vi "Write Name.vi"(10 "Name":string, 11 "Person In":refnum<class "Person.lvclass">) -> (3 "Person Out":refnum<class "Person.lvclass">)   [LabVIEW 2018, in "Person.lvclass"]
uses:
  Person.lvclass
  Person.lvclass/Person.ctl
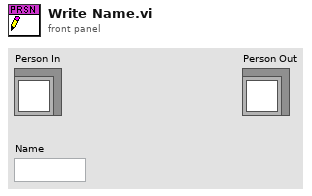
[diagram p1: front panel]
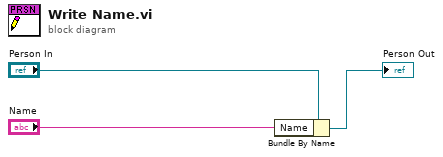
[diagram p0: block diagram]
diagram:
  n1 = Bundle By Name(cluster="Person In", "Name"="Name") -> (→"Person Out":refnum<class "Person.lvclass">)
